vi "Init_Instr.vi"(8 "error in (no error)":errorcluster caption="entrée d'erreur (pas d'erreur)", 11 "Class Instrument Process en entrée":refnum<class "Class Instrument Process.lvclass">) -> (0 "error out":errorcluster caption="sortie d'erreur", 3 "Class Instrument Process en sortie":refnum<class "Class Instrument Process.lvclass">)   [LabVIEW 2020, in "Library Instrument & Equipement.lvlib" / "Library Instruments.lvlib" / "Class Instrument Process.lvclass"]
uses:
  Class Instrument Process.lvclass
  Class Instrument Process.lvclass/Class Instrument Process.ctl
  Instrument (Default)/Class Instrument (Default).lvclass
  Process/Process (Default)/Process (Default).lvclass
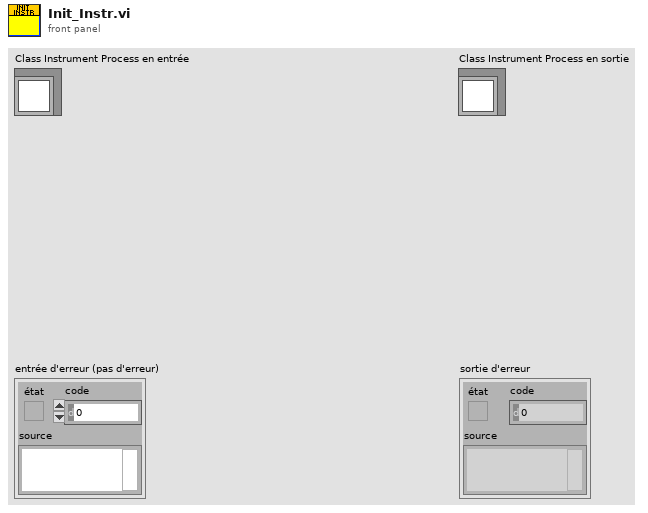
[diagram p1: front panel]
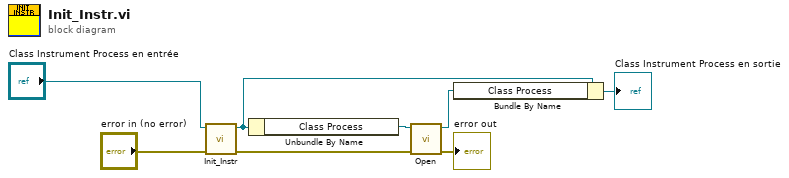
[diagram p0: block diagram]
diagram:
  n1 = call-parent "Init_Instr.vi"("error in (no error)"="error in (no error)", "Class Instrument (Default) en entrée"="Class Instrument Process en entrée") -> ("error out"=w3:errorcluster, "Class Instrument (Default) en sortie"=w5:refnum<class "Class Instrument Process.lvclass">)  [unwired: 8 in]
  n2 = Unbundle By Name(w5) -> ("Class Process"=w4:refnum<class "Process (Default).lvclass">)
  n3 = call-dynamic "Open.vi"("error in (no error)"=w3, "Process (Default) en entrée"=w4) -> ("error out"=→"error out":errorcluster, "Process (Default) en sortie"=w1:refnum<class "Process (Default).lvclass">)  [unwired: 8 in]
  n4 = Bundle By Name(cluster=w5, "Class Process"=w1) -> (→"Class Instrument Process en sortie":refnum<class "Class Instrument Process.lvclass">)
